vi "WirtePackageData.vi"() -> ()   [LabVIEW 2013]
panel:
  out "ReportStrA":string
  in  "SendAD":string
  in  "BoxNo":string
  in  "PartNum":string
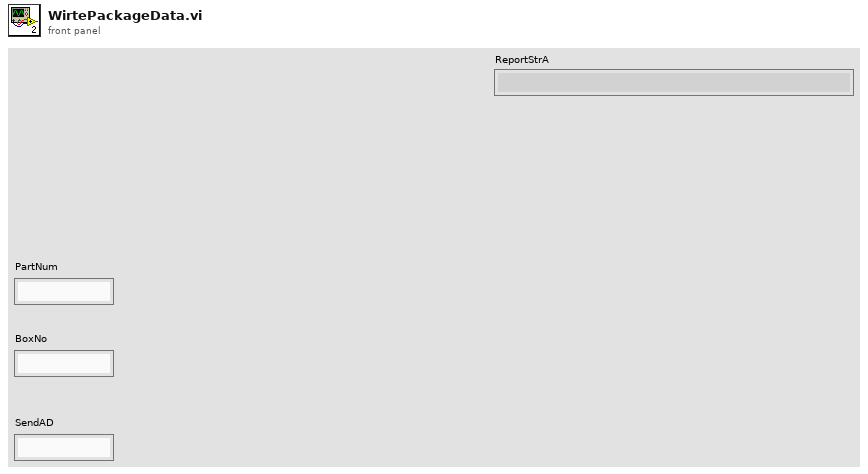
[diagram p1: front panel]
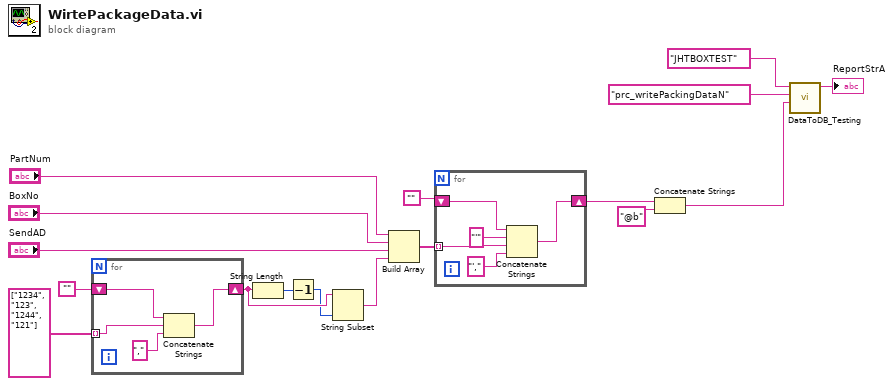
[diagram p0: block diagram]
diagram:
  n1 = for {
    shift-right: [w20] -> w12
    shift-left: "" -> [w21]
    tunnel: string[] ["1234", "123", "1244", "121"] -> [w19] mode=indexing
    n2 = Concatenate Strings(w21, w19, "," ("SendAD 2")) -> (w20:string)
  }
  n3 = String Length(string=w12) -> (length=w13:i32)
  n4 = Decrement(x=w13) -> (x-1=w11:i32)
  n5 = String Subset(string=w12, length (rest)=w11) -> (substring=w4:string)  [unwired: 1 in]
  n6 = Build Array("PartNum", "BoxNo", "SendAD", w4) -> (w5:string[])
  n7 = for {
    shift-right: [w25] -> w10
    shift-left: "" -> [w26]
    tunnel: w5 -> [w22] mode=indexing
    n8 = Concatenate Strings(w26, "'" ("SendAD 2"), w22, "'," ("SendAD 2")) -> (w25:string)
  }
  n9 = Concatenate Strings(w10, "@b") -> (w2:string)
  n10 = call "DataToDB_Testing.vi"("all string"=w2, "Procedure name"="prc_writePackingDataN", "DSN name"="JHTBOXTEST") -> ("ReportStrA"=→"ReportStrA":string)  [unwired: 7 in, 1 out]
